vi "Start activity (subVi).vi"(2 "error in":errorcluster, 3 "Text Ring":u16(ring) items=["Filament off/Saving off", "Filament on/Saving off", "Filament on/Saving on"]) -> (0 "error out":errorcluster)   [LabVIEW 2016]
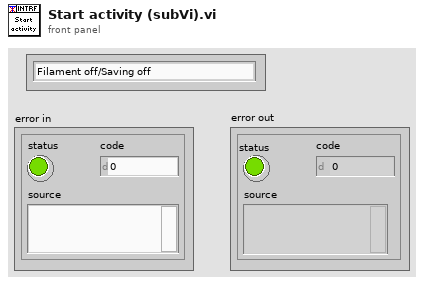
[diagram p1: front panel]
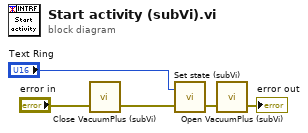
[diagram p0: block diagram]
diagram:
  n1 = call "Close VacuumPlus (subVi).vi"("error in (no error)"="error in") -> ("error out"=w4:errorcluster)  [unwired: 1 in, 1 out]
  n2 = call "Set state (subVi).vi"("error in"=w4, "Text Ring"="Text Ring") -> ("error out"=w5:errorcluster)  [unwired: 1 in]
  n3 = call "Open VacuumPlus (subVi).vi"("error in (no error)"=w5) -> ("error out"=→"error out":errorcluster)  [unwired: 1 in, 1 out]
